vi "Preview.vi"(8 "error in (no error)":errorcluster, 11 "VI View in":refnum<class "VI View.lvclass">) -> (0 "error out":errorcluster, 3 "VI View out":refnum<class "VI View.lvclass">)   [LabVIEW 2013, in "SET Project Editor.lvlib" / "VI View.lvclass"]
uses:
  VI View.lvclass
  VI View.lvclass/VI View.ctl
  SET Project Data/VI Class/VI Data.lvclass
  SET Project Data/VI Class/Read Languages.vi
  SET Project Editor.lvlib
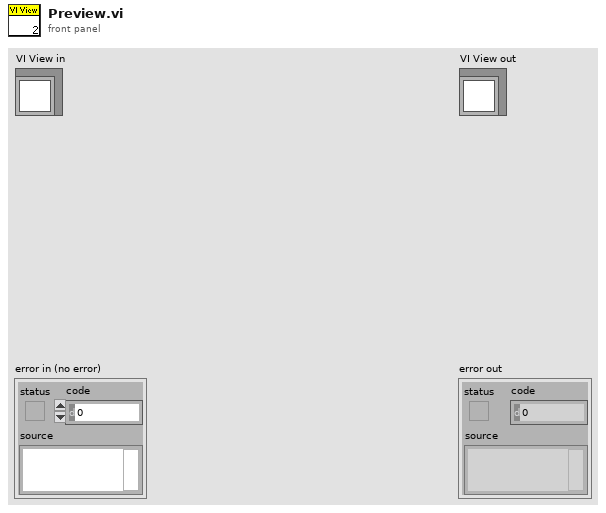
[diagram p1: front panel]
types:
  T1 = typedef "SET Resource File.lvlib/ResFile Lang Entry.ctl" = cluster{"Tag":string, "Name":string, "Code Page":u16}
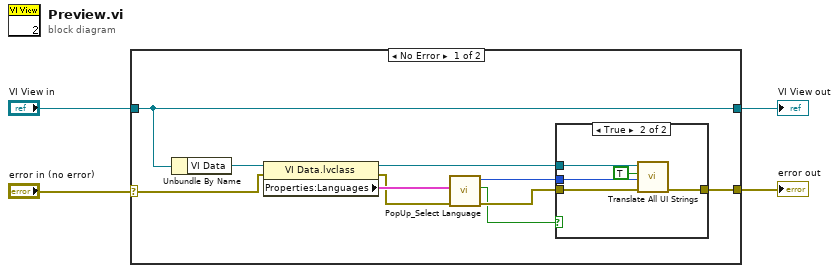
[diagram p0: block diagram]
diagram:
  n1 = case shown="No Error" "error in (no error)" {
    selector: "error in (no error)" -> [w6 w22]
    tunnel: [w5 w22] -> w3
    tunnel: [w14 w21] -> w1
    tunnel: "VI View in" -> [w14 w21]
    frame No Error {
      n2 = Unbundle By Name(w14) -> ("VI Data"=w13:refnum<class "VI Data.lvclass">)
      n3 = property class="VI Data.lvclass"(reference=w13, error in=w6) -> (reference out=w12:refnum<class "VI Data.lvclass">, error out=w10:errorcluster, "Properties:Languages"=w11:T1[])
      n4 = call "PopUp_Select Language.vi"("error in (no error)"=w10, "Languages"=w11) -> ("error out"=w9:errorcluster, "OK Pressed?"=w7:bool, "LangIndex"=w8:i32)  [unwired: 7 in]
      n5 = case shown="True" w7 {
        tunnel: w12 -> [_ w18]
        tunnel: w9 -> [w15 w17]
        tunnel: w8 -> [_ w20]
        tunnel: [w15 w19] -> w5
        frame False {
        }
        frame True {
          n6 = call-dynamic "Translate All UI Strings.vi"("error in (no error)"=w17, "Language Index (0)"=w20, "Preview?"=TRUE, "LanguageData in"=w18) -> ("error out"=w19:errorcluster)  [unwired: 6 in, 1 out]
        }
      }
    }
    frame Error {
    }
  }
  "error out" <- w3
  "VI View out" <- w1
